vi "ChargeBanks.vi"(9 "Abort":refnum<vi>, 10 "Experiment State":T1={"Send Trigger 3"=FALSE, "error"={"status"=FALSE, "code"=0, "source"=""}, "Tasks"={"Fiber15 MP Task"="MyVoltageTask", "Read Slow AI"="", "Fiber Bank DIO"="", "Fiber7 MP Task"="MyVoltageTask", "TaskArray"=[]}, "Channels"={"6133 Channels"=[], "Trigger Source"="", "Edge Type"=10280, "Samples Per Channel"=[], "#Pre-Trigger Samples"=[], "Sample Rate 2.5Ms/s Max"=[]}, "Dev 10 DIO"="", "Dev5"="", "Fiber Triggers 2"=[{"Delay (s)"=2.559999942779541, "Pulse width (s)"=0.009999999776482582, "Active"=TRUE, "Channel Name"="Fiber 8", "counter"="PXI1Slot8/ctr7"}], "MP7"=FALSE, "MP15"=FALSE, "PXI Slot 2"={"PXI Slot 2 Handle"="PXI1Slot2", "source terminal"="GlobalSoftwareTrigger"}, "# of Control DIOs"=0, "Bank DIO Settings"=[], "Purge Duration (s)"=5, "Interlock Override"=FALSE, "Current Raw Voltages, Slot &"=[], "Bank Control"={"Bank Enables"={"Gun1 Enable"=FALSE, "Gun2 Enable"=FALSE, "InnerSol Enable"=FALSE, "OuterSol1 Enable"=FALSE, "Outer2 Enable"=FALSE, "Gun3 Enable"=FALSE}, "Voltages"={"Gun1 Voltage"=0.0, "Gun2 Voltage"=0.0, "Gun3 Voltage"=0.0, "InnerSol Voltage"=0.0, "OuterSol1 Voltage"=0.0, "OuterSol2 Voltage"=0.0}, "Set Points"={"Gun1 Setpoint"=0.0, "Gun2 Setpoint"=0.0, "Gun3 Setpoint"=0.0, "InnerSol Setpoint"=0.0, "OuterSol1 Setpoint"=0.0, "OuterSol2 Setpoint"=0.0}}, "Waveform Data"=[], "Next Shot#"="0", "Slot 7, Last Shot Scaled Voltages"=[], "Data Run Description"="", "Next Shot Data"=["599", "6/18/2009", "4:08PM", "Ziemba", "Bank Testing", "-7.142518", "-8.256295", "-6.893030", "-5.120022", "-0.001235", "-0.001559", "-0.000910", "-0.001235", "-0.001235", "-0.001235", "-0.001235", "0.114909", "-0.000586", "-0.000586", "0.684598", "1.197512"], "Headers"=[], "Html Shot Log View"=FALSE, "ShotLog Headers"=path "", "ShotLog Data"=path "", "Enable Bank Control"=FALSE, "6602  Slot8"={"Slot 8 Trigger Source"="", "Slot 8 Clock Source"="", "Trigger Channel Tasks"=[]}, "6602  Slot 9"={"Slot 9 Clock Source"="", "Slot 9 Trigger Source"="", "Trigger Channel Tasks"=[]}, "Total Sample Time (us)"=[], "Pre-Trigger Time (us)"=[], "Fiber Triggers"=[{"Delay (s)"=2.559999942779541, "Pulse width (s)"=0.009999999776482582, "Active"=TRUE, "Channel Name"="ns", "counter"=""}], "System Message"=""} {"Fiber Triggers"."Pulse width (s)" format="%.3p"; "Fiber Triggers"."Delay (s)" format="%.3p"; "Pre-Trigger Time (us)" format="%#_6f"; "Total Sample Time (us)" format="%#_6f"; "Current Raw Voltages, Slot &" format="%0.2f"; "Fiber Triggers 2"."Pulse width (s)" format="%.3p"; "Fiber Triggers 2"."Delay (s)" format="%.3p"; "Channels"."Sample Rate 2.5Ms/s Max" format="%#_3p"; "Channels"."Edge Type" items=["Rising"=10280, "Falling"=10171]}, 11 "Bank Charge":refnum<vi>) -> (2 "Experiment State":T1={"Send Trigger 3"=FALSE, "error"={"status"=FALSE, "code"=0, "source"=""}, "Tasks"={"Fiber15 MP Task"="MyVoltageTask", "Read Slow AI"="", "Fiber Bank DIO"="", "Fiber7 MP Task"="MyVoltageTask", "TaskArray"=[]}, "Channels"={"6133 Channels"=[], "Trigger Source"="", "Edge Type"=10280, "Samples Per Channel"=[], "#Pre-Trigger Samples"=[], "Sample Rate 2.5Ms/s Max"=[]}, "Dev 10 DIO"="", "Dev5"="", "Fiber Triggers 2"=[{"Delay (s)"=2.559999942779541, "Pulse width (s)"=0.009999999776482582, "Active"=TRUE, "Channel Name"="Fiber 8", "counter"="PXI1Slot8/ctr7"}], "MP7"=FALSE, "MP15"=FALSE, "PXI Slot 2"={"PXI Slot 2 Handle"="PXI1Slot2", "source terminal"="GlobalSoftwareTrigger"}, "# of Control DIOs"=0, "Bank DIO Settings"=[], "Purge Duration (s)"=5, "Interlock Override"=FALSE, "Current Raw Voltages, Slot &"=[], "Bank Control"={"Bank Enables"={"Gun1 Enable"=FALSE, "Gun2 Enable"=FALSE, "InnerSol Enable"=FALSE, "OuterSol1 Enable"=FALSE, "Outer2 Enable"=FALSE, "Gun3 Enable"=FALSE}, "Voltages"={"Gun1 Voltage"=0.0, "Gun2 Voltage"=0.0, "Gun3 Voltage"=0.0, "InnerSol Voltage"=0.0, "OuterSol1 Voltage"=0.0, "OuterSol2 Voltage"=0.0}, "Set Points"={"Gun1 Setpoint"=0.0, "Gun2 Setpoint"=0.0, "Gun3 Setpoint"=0.0, "InnerSol Setpoint"=0.0, "OuterSol1 Setpoint"=0.0, "OuterSol2 Setpoint"=0.0}}, "Waveform Data"=[], "Next Shot#"="0", "Slot 7, Last Shot Scaled Voltages"=[], "Data Run Description"="", "Next Shot Data"=["599", "6/18/2009", "4:08PM", "Ziemba", "Bank Testing", "-7.142518", "-8.256295", "-6.893030", "-5.120022", "-0.001235", "-0.001559", "-0.000910", "-0.001235", "-0.001235", "-0.001235", "-0.001235", "0.114909", "-0.000586", "-0.000586", "0.684598", "1.197512"], "Headers"=[], "Html Shot Log View"=FALSE, "ShotLog Headers"=path "", "ShotLog Data"=path "", "Enable Bank Control"=FALSE, "6602  Slot8"={"Slot 8 Trigger Source"="", "Slot 8 Clock Source"="", "Trigger Channel Tasks"=[]}, "6602  Slot 9"={"Slot 9 Clock Source"="", "Slot 9 Trigger Source"="", "Trigger Channel Tasks"=[]}, "Total Sample Time (us)"=[], "Pre-Trigger Time (us)"=[], "Fiber Triggers"=[{"Delay (s)"=2.559999942779541, "Pulse width (s)"=0.009999999776482582, "Active"=TRUE, "Channel Name"="ns", "counter"=""}], "System Message"=""} {"Fiber Triggers"."Pulse width (s)" format="%.3p"; "Fiber Triggers"."Delay (s)" format="%.3p"; "Pre-Trigger Time (us)" format="%#_6f"; "Total Sample Time (us)" format="%#_6f"; "Current Raw Voltages, Slot &" format="%0.2f"; "Fiber Triggers 2"."Pulse width (s)" format="%.3p"; "Fiber Triggers 2"."Delay (s)" format="%.3p"; "Channels"."Sample Rate 2.5Ms/s Max" format="%#_3p"; "Channels"."Edge Type" items=["Rising"=10280, "Falling"=10171]})   [LabVIEW 2013]
uses:
  Controls/ExperimentStateCluster.ctl
  <vilib>/Platform/TimedLoop/XDataNode/timing_clust.ctl
  <vilib>/Platform/TimedLoop/XDataNode/nitl_modes.ctl
  <vilib>/Platform/TimedLoop/XDataNode/wakeup.ctl
  <vilib>/DAQmx/read.llb/DAQmx Read (Analog 2D DBL NChan NSamp).vi
  <vilib>/DAQmx/write.llb/DAQmx Write (Digital 1D Bool NChan 1Samp 1Line).vi
  <vilib>/DAQmx/miscellaneous.llb/DAQmx Fill In Error Info.vi
  <vilib>/platform/TimedLoop/XDataNode/XDataNode.xnode
  <vilib>/Platform/TimedLoop/XDataNode/XDNodeRunTimeDep.lvlib
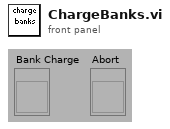
[diagram p1: front panel]
types:
  T1 = typedef "ExperimentStateCluster.ctl" = cluster{"Send Trigger 3":bool, "error":errorcluster, "Tasks":cluster{"Fiber15 MP Task":refnum<k21>, "Read Slow AI":refnum<k21>, "Fiber Bank DIO":refnum<k21>, "Fiber7 MP Task":refnum<k21>, "TaskArray":refnum<k21>[]}, "Channels":cluster{"6133 Channels":tag[], "Trigger Source":tag, "Edge Type":i32, "Samples Per Channel":i32[], "#Pre-Trigger Samples":u32[], "Sample Rate 2.5Ms/s Max":dbl[]}, "Dev 10 DIO":refnum<k21>, "Dev5":refnum<k21>, "Fiber Triggers 2":cluster{"Delay (s)":dbl, "Pulse width (s)":dbl, "Active":bool, "Channel Name":string, "counter":tag}[], "MP7":bool, "MP15":bool, "PXI Slot 2":cluster{"PXI Slot 2 Handle":refnum<k15>, "source terminal":string}, "# of Control DIOs":i32, "Bank DIO Settings":bool[], "Purge Duration (s)":u32, "Interlock Override":bool, "Current Raw Voltages, Slot &":dbl[], "Bank Control":cluster{"Bank Enables":cluster{"Gun1 Enable":bool, "Gun2 Enable":bool, "InnerSol Enable":bool, "OuterSol1 Enable":bool, "Outer2 Enable":bool, "Gun3 Enable":bool}, "Voltages":cluster{"Gun1 Voltage":dbl, "Gun2 Voltage":dbl, "Gun3 Voltage":dbl, "InnerSol Voltage":dbl, "OuterSol1 Voltage":dbl, "OuterSol2 Voltage":dbl}, "Set Points":cluster{"Gun1 Setpoint":dbl, "Gun2 Setpoint":dbl, "Gun3 Setpoint":dbl, "InnerSol Setpoint":dbl, "OuterSol1 Setpoint":dbl, "OuterSol2 Setpoint":dbl}}, "Waveform Data":waveform(dbl)[][], "Next Shot#":string, "Slot 7, Last Shot Scaled Voltages":string[], "Data Run Description":string, "Next Shot Data":string[], "Headers":string[], "Html Shot Log View":bool, "ShotLog Headers":path, "ShotLog Data":path, "Enable Bank Control":bool, "6602  Slot8":cluster{"Slot 8 Trigger Source":tag, "Slot 8 Clock Source":tag, "Trigger Channel Tasks":refnum<k21>[]}, "6602  Slot 9":cluster{"Slot 9 Clock Source":tag, "Slot 9 Trigger Source":tag, "Trigger Channel Tasks":refnum<k21>[]}, "Total Sample Time (us)":dbl[], "Pre-Trigger Time (us)":dbl[], "Fiber Triggers":cluster{"Delay (s)":dbl, "Pulse width (s)":dbl, "Active":bool, "Channel Name":string, "counter":tag}[], "System Message":string}
  T2 = typedef "XDNodeRunTimeDep.lvlib/timing_clust.ctl" = cluster{"Expected End [f-1]":u64, "Actual End [f-1]":u64, "Finished Late? [f-1]":bool, "Expected End [i-1]":u64, "Actual End [i-1]":u64, "Finished Late? [i-1]":bool, "Expected Start [i]":u64, "Actual Start [i]":u64, "Expected Start [f]":u64, "Actual Start [f]":u64, "Source Name":string, "Structure Name":string, "Period":i64, "Deadline":i64, "Offset":i64, "Start":i64, "Priority":i32, "Timeout":i32, "Mode":T3, "Wakeup Reason":T4, "Error":errorcluster, "Source Type":string, "Secondary Source Type":string, "Global End Time":u64, "Global Start Time":u64, "Frame Duration":u64, "Iteration Duration":u64, "Assigned CPU":i32, "I/O Scan Engine Mode":u32}
  T3 = typedef "XDNodeRunTimeDep.lvlib/nitl_modes.ctl" = enum32{"No Change", "Process missed periods, maintain original phase", "Discard missed periods, maintain original phase", "Process missed periods, ignore original phase", "Discard missed periods, ignore original phase"}
  T4 = typedef "XDNodeRunTimeDep.lvlib/wakeup.ctl" = enum32{"Normal", "Aborted", "Asynchronous wakeup", "Timing source error", "Timed loop error", "Timeout"}
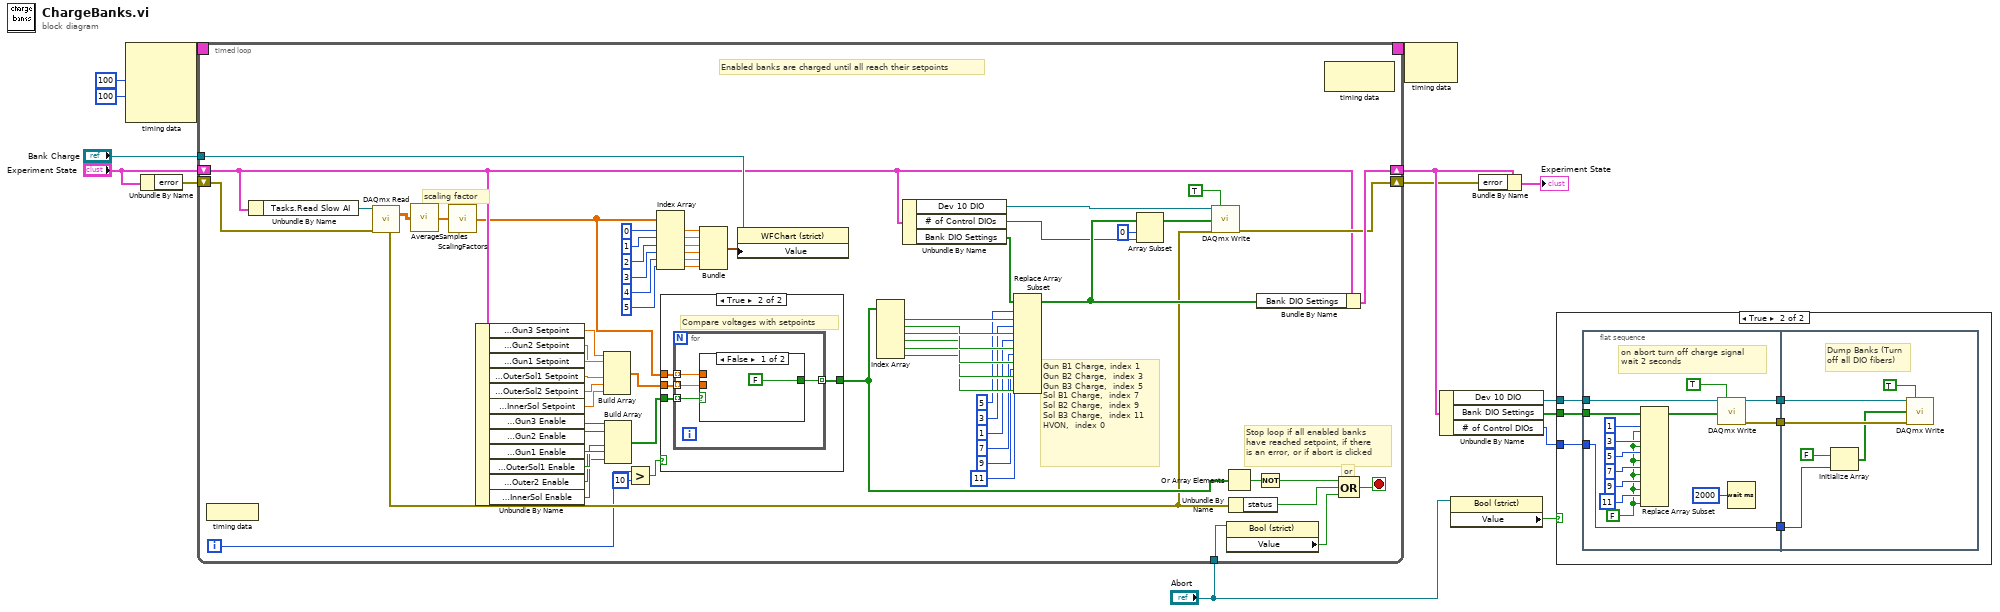
[diagram p0: block diagram]
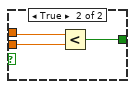
[diagram p4: hidden frame]
diagram:
  n1 = node-c288(i64 100 ("Period"), 100 ("Priority")) -> (w15:T2)  [unwired: 2 out]
  n2 = Unbundle By Name("Experiment State") -> ("error"=w5:errorcluster)
  n3 = timed-loop {
    timing: w15 -> [_]
    timing-out: [_] -> w14
    shift-right: [w69] -> w3
    shift-left: "Experiment State" -> [w42]
    tunnel: "Bank Charge" -> [w49]
    tunnel: "Abort" -> [w67]
    shift-right: [w47] -> w2
    shift-left: w5 -> [w46]
    i -> [w35]
    stop <- w48 stop-if-true
    # "scaling factor"
    # "Stop loop if all enabled banks\nhave reached setpoint, if there\nis an error, or if abort is clicked"
    # "Enabled banks are charged until all reach their setpoints"
    # "or"
    # "Gun B1 Charge, index 1\nGun B2 Charge,  index 3\nGun B3 Charge,  index 5 \nSol B1 Charge,  index 7\nSol B2 Charge,  index 9\nSol B3 Charge,  index 11\nHVON,  index 0"
    n4 = node-c288() -> ()  [unwired: 1 out]
    n5 = Unbundle By Name(w42) -> ("Tasks.Read Slow AI"=w68:refnum<k21>)
    n6 = call-poly <vilib>:"DAQmx Read.vi"("task/channels in"=w68, "error in"=w46) -> ("data"=w25:dbl[][], "error out"=w45:errorcluster)  [unwired: 1 in, 11 out]
    n7 = call "AverageSamples.vi"("data"=w25) -> ("Array"=w24:dbl[])
    n8 = call "ScalingFactors.vi"("Input measurements"=w24) -> ("Output measurements"=w23:dbl[])
    n9 = Unbundle By Name(w42) -> ("Bank Control.Set Points.Gun3 Setpoint"=w17:dbl, "Bank Control.Set Points.Gun2 Setpoint"=w18:dbl, "Bank Control.Set Points.Gun1 Setpoint"=w19:dbl, "Bank Control.Set Points.OuterSol1 Setpoint"=w20:dbl, "Bank Control.Set Points.OuterSol2 Setpoint"=w21:dbl, "Bank Control.Set Points.InnerSol Setpoint"=w22:dbl, "Bank Control.Bank Enables.Gun3 Enable"=w32:bool, "Bank Control.Bank Enables.Gun2 Enable"=w31:bool, "Bank Control.Bank Enables.Gun1 Enable"=w30:bool, "Bank Control.Bank Enables.OuterSol1 Enable"=w29:bool, "Bank Control.Bank Enables.Outer2 Enable"=w28:bool, "Bank Control.Bank Enables.InnerSol Enable"=w27:bool)
    n10 = Build Array(w17, w18, w19, w20, w21, w22) -> (w16:dbl[])
    n11 = Build Array(w32, w31, w30, w29, w28, w27) -> (w26:bool[])
    n12 = Greater?(x=w35, y=10) -> (0:w33:bool)
    n13 = Index Array(array=w23, index #1=0 ("index"), index #2=1 ("index"), index #3=2 ("index"), index #4=3 ("index"), index #5=4 ("index"), index #6=5 ("index")) -> (element #1=w59:dbl, element #2=w58:dbl, element #3=w57:dbl, element #4=w56:dbl, element #5=w55:dbl, element #6=w54:dbl)
    n14 = case shown="True" w33 {
      tunnel: w16 -> [_ w86]
      tunnel: w26 -> [w82 w85]
      tunnel: [w82 w84] -> w64
      tunnel: w23 -> [_ w83]
      frame False {
        # "Keep charge on for first few \niterations to ignore transient\nvoltages from relays"
      }
      frame True {
        # "Compare voltages with setpoints"
        n15 = for {
          tunnel: w83 -> [w90] mode=indexing
          tunnel: w86 -> [w89] mode=indexing
          tunnel: w85 -> [w88] mode=indexing
          tunnel: [w87] -> w84 mode=indexing
          n16 = case shown="False" w88 {
            tunnel: w90 -> [_ w93]
            tunnel: w89 -> [_ w94]
            tunnel: [FALSE w92] -> w87
            frame False {
            }
            frame True {
              n17 = Less?(x=w93, y=w94) -> (x < y?=w92:bool)
            }
          }
        }
      }
    }
    n18 = Bundle(w59, w58, w57, w56, w55, w54) -> (w50:cluster{dbl, dbl, dbl, dbl, dbl, dbl})  [unwired: 1 in]
    n19 = property on="Property Node" class="WFChart (strict)"(reference=w49, "Value"=w50) -> ()  [unwired: 1 in, 2 out]
    n20 = Index Array(array=w64) -> (element #1=w75:bool, element #2=w74:bool, element #3=w73:bool, element #4=w72:bool, element #5=w71:bool, element #6=w70:bool)  [unwired: 6 in]
    n21 = Unbundle By Name(w42) -> ("Dev 10 DIO"=w43:refnum<k21>, "# of Control DIOs"=w63:i32, "Bank DIO Settings"=w77:bool[])
    n22 = Replace Array Subset(array=w77, new element #1=w75, index #1=5 ("index"), new element #2=w74, index #2=3 ("index"), new element #3=w73, index #3=1 ("index"), new element #4=w72, index #4=7 ("index"), new element #5=w71, index #5=9 ("index"), new element #6=w70, index #6=11 ("index")) -> (w76:bool[])
    n23 = Array Subset(array=w76, index=0, length=w63) -> (w78:bool[])
    n24 = call-poly <vilib>:"DAQmx Write.vi"("task/channels in"=w43, "auto start"=TRUE, "data"=w78, "error in"=w45) -> ("error out"=w47:errorcluster)  [unwired: 11 out]
    n25 = Or Array Elements(Boolean array=w64) -> (logical OR=w81:bool)
    n26 = property class="Bool (strict)"(reference=w67) -> ("Value"=w65:bool)  [unwired: 1 in, 2 out]
    n27 = Unbundle By Name(w45) -> ("status"=w44:bool)
    n28 = Bundle By Name(cluster=w42, "Bank DIO Settings"=w76) -> (w69:T1)
    n29 = Not(x=w81) -> (.not. x?=w66:bool)
    n30 = node-c288() -> ()  [unwired: 2 out]
    n31 = Compound Arithmetic op=OR(w66, w44, w65) -> (w48:bool)
  }
  n32 = node-c288(w14) -> ()  [unwired: 1 out]
  n33 = Unbundle By Name(w3) -> ("Dev 10 DIO"=w8:refnum<k21>, "Bank DIO Settings"=w1:bool[], "# of Control DIOs"=w7:i32)
  n34 = property class="Bool (strict)"(reference="Abort") -> ("Value"=w9:bool)  [unwired: 1 in, 2 out]
  n35 = Bundle By Name(cluster=w3, "error"=w2) -> (→"Experiment State":T1)
  n36 = case shown="True" w9 {
    tunnel: w8 -> [_ w102]
    tunnel: w7 -> [_ w101]
    tunnel: w1 -> [_ w100]
    frame False {
    }
    frame True {
      n37 = flat-sequence {
        tunnel: w102 -> [w117]
        tunnel: w101 -> [w103]
        tunnel: w100 -> [w114]
        tunnel: [w105] -> w99
        tunnel: [w104] -> w98
        tunnel: [w103] -> w97
        tunnel: w99 -> [w123]
        tunnel: w98 -> [w122]
        tunnel: w97 -> [w120]
        frame #0 {
          w106 = FALSE ("new element/subarray")
          # "on abort turn off charge signal\nwait 2 seconds"
          n38 = Replace Array Subset(array=w114, new element #1=w106, index #1=1 ("index"), new element #2=w106, index #2=3 ("index"), new element #3=w106, index #3=5 ("index"), new element #4=w106, index #4=7 ("index"), new element #5=w106, index #5=9 ("index"), new element #6=w106, index #6=11 ("index")) -> (w113:bool[])
          n39 = call-poly <vilib>:"DAQmx Write.vi"("task/channels in"=w117, "auto start"=TRUE, "data"=w113) -> ("task out"=w105:refnum<k21>, "error out"=w104:errorcluster)  [unwired: 2 in, 9 out]
          n40 = Wait (ms)(milliseconds to wait=u32 2000) -> ()  [unwired: 1 out]
        }
        frame #1 {
          # "Dump Banks (Turn off all DIO fibers)"
          n41 = Initialize Array(FALSE ("new element/subarray"), w120) -> (w119:bool[])
          n42 = call-poly <vilib>:"DAQmx Write.vi"("task/channels in"=w123, "auto start"=TRUE, "data"=w119, "error in"=w122) -> ()  [unwired: 1 in, 11 out]
        }
      }
    }
  }
